vi "Ex8.vi"() -> ()   [LabVIEW 2016]
panel:
  out "웨이브폼 그래프":i32[](graph)
  out "웨이브폼 차트":i32(graph)
  # "여러번 이 VI를 실행하면, 차트는 원래 있는 값에서 \n계속 적으로 값이 쌓이고 있는 것을 \n발견할 수 있습니다. 반대로, 그래프는 매번 전에 \n있던 데이터는 초기화 되고 한번에 그려지는 것을 \n확인할 수 있습니다.\n\n차트에서는 값이 계속 적으로 쌓이기 때문에 \n원소를 입력값으로 써서 전에 있던 데이터 라인에 \n더해집니다. 과거의 데이터를 저장 하는데에 있어 \n일정 메모리가 할당 됩니다.\n\n반면에 그래프경우, 전의 값들은 초기화가 되고, \n한번에 값이 들어가야 하는 이유로 입력값으로\n원소를 넣을 수 없고, 배열 이상의 값을 넣어야 합니다.\n과거의 데이터를 저장 할 필요가 없어 추가적\n메모리를 요구하지 않습니다."
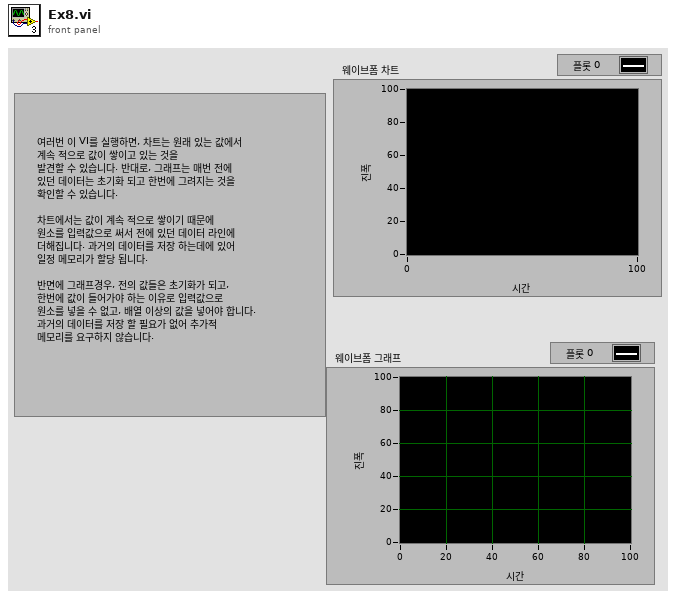
[diagram p1: front panel]
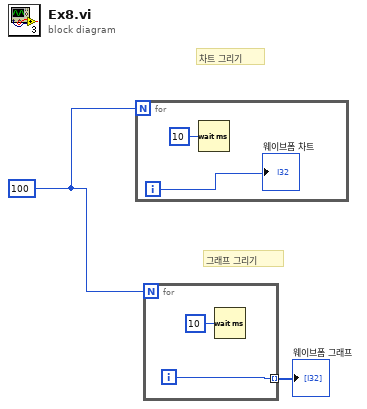
[diagram p0: block diagram]
diagram:
  w2 = 100
  # "그래프 그리기"
  # "차트 그리기"
  n1 = for {
    N: w2 -> [_]
    i -> [w3]
    n2 = Wait (ms)(milliseconds to wait=u32 10 ("대기 시간 (ms)")) -> ()  [unwired: 1 out]
    "웨이브폼 차트" <- w3
  }
  n3 = for {
    N: w2 -> [_]
    tunnel: [w6] -> w1 mode=indexing
    i -> [w6]
    n4 = Wait (ms)(milliseconds to wait=u32 10 ("대기 시간 (ms)")) -> ()  [unwired: 1 out]
  }
  "웨이브폼 그래프" <- w1
